vi "Read Analog Input Values.vi"(8 "error in":errorcluster, 9 "Timeout / s":dbl=10.0 format="%0.2f", 10 "AI ULx Task":refnum<k24>, 11 "BNT_ULx-MCSV in":refnum<class "BNT_ULx-MCSV.lvclass">) -> (0 "error out":errorcluster, 1 "AI Data":dbl[](array[numeric]), 3 "BNT_ULx-MCSV out":refnum<class "BNT_ULx-MCSV.lvclass">)   [LabVIEW 2020, in "BNT_ULx.lvlib" / "BNT_ULx-MCSV.lvclass"]
doc: "Read analog input.\n\n<b>Default Implementation:</b> Analog Input\n\nThis dynamic dispatch VI can be overritten by derived classes to implement other analog input readings."
uses:
  BNT_ULx-MCSV.lvclass
  <vilib>/DAQmx/miscellaneous.llb/DAQmx Fill In Error Info.vi
  BNT_ULx-MCSV.lvclass/BNT_ULx-MCSV.ctl
  <vilib>/ULx/Read.llb/ULx Read (Analog 1D DBL NChan 1Samp).vi
  C:/Program Files (x86)/National Instruments/LabVIEW 2020/vi.lib/ULx/ULx_LV.dll
  Program Files (x86)/National Instruments/LabVIEW 2020/vi.lib/ULx/ULx_LV.dll
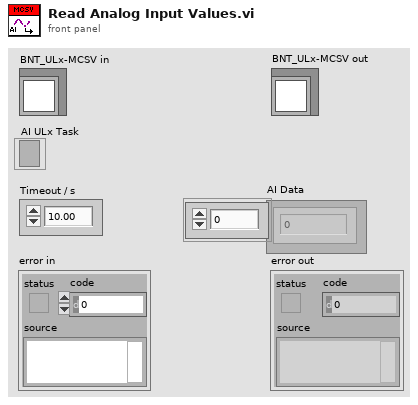
[diagram p1: front panel]
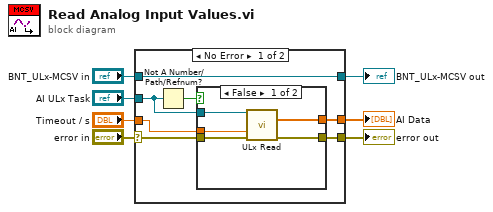
[diagram p0: block diagram]
diagram:
  n1 = case shown="No Error" "error in" {
    selector: "error in" -> [w13 w22]
    tunnel: [w12 w22] -> w6
    tunnel: [w10 w21] -> w4
    tunnel: "BNT_ULx-MCSV in" -> [w10 w21]
    tunnel: "Timeout / s" -> [w14 _]
    tunnel: [w11 _] -> w2
    tunnel: "AI ULx Task" -> [w8 _]
    frame No Error {
      n2 = Not A Number/Path/Refnum?(number/path/refnum=w8) -> (NaN/Path/Refnum?=w9:bool)
      n3 = case shown="False" w9 {
        tunnel: w14 -> [w15 _]
        tunnel: w13 -> [w18 w20]
        tunnel: [w19 w20] -> w12
        tunnel: [w16 _] -> w11
        tunnel: w8 -> [w17 _]
        frame False {
          n4 = call-poly <vilib>:"ULx Read.vi"("task in"=w17, "timeout"=w15, "error in"=w18) -> ("data"=w16:dbl[], "error out"=w19:errorcluster)  [unwired: 10 in, 1 out]
        }
        frame True {
        }
      }
    }
    frame Error {
    }
  }
  "error out" <- w6
  "BNT_ULx-MCSV out" <- w4
  "AI Data" <- w2
